vi "Get_RegData_TypeString.vi"(8 "error in (no error)":errorcluster, 11 "RegData_I32 in":refnum<class "IB_RegData_I32.lvclass">) -> (0 "error out":errorcluster, 2 "Type String":string, 3 "RegData_I32 out":refnum<class "IB_RegData_I32.lvclass">)   [LabVIEW 2020, in "IB_RegData_I32.lvclass"]
uses:
  <vilib>/AppBuilder/IB_Classes/RegData/RegData_I32/IB_RegData_I32.lvclass
  <vilib>/AppBuilder/IB_Classes/RegData/RegData_I32/IB_RegData_I32.lvclass/IB_RegData_I32.ctl
  <resource>/Framework/Providers/Builds/Installer/CDK_GLOBAL_STRINGS.vi
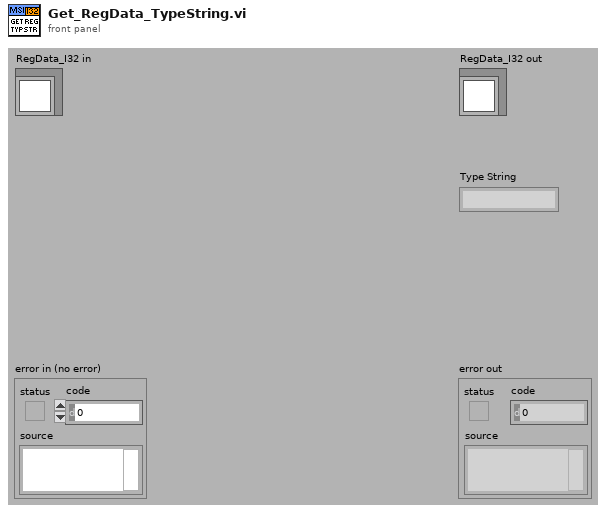
[diagram p1: front panel]
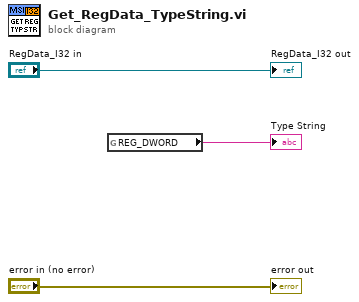
[diagram p0: block diagram]
diagram:
  n1 = global read "CDK_GLOBAL_STRINGS.vi" "REG_DWORD"() -> (→"Type String":string)
  "error out" <- "error in (no error)"
  "RegData_I32 out" <- "RegData_I32 in"
